vi "Bertta_v09_93.vi"() -> ()   [LabVIEW 2015]
panel:
  out "element":bool
  out "Started:":string
  in  "SHUTDOWN":bool
  in  "MASTER CONTROL":bool
  in  "Tab Control":T1(tab)
  out "Output File":path caption="selected path"
  in  "Browse folder":path=path "" caption="start path"
  in  "Read Seq":bool
  in  "Save Seq":bool
  in  "Configuration file":path=path "C:/Users/shresplab/Desktop/BerttaConfiguration.lvm" caption="Filename"
  in  "OK Button 2":bool
  out "Boolean":bool
  in  "User (initials)":string
  in  "Project name":string
  in  "Description":string
  out "PUMP1":bool
  out "Target amount":dbl
  out "Scale weight":dbl
  out "Amount now":dbl
  out "Flow rate":dbl
  out "Time to target":dbl format="%<%H:%M:%S>t"
  out "Current step":dbl
  out "Target":dbl
  out "Amount now":dbl
  out "Amount now":dbl
  out "Target":dbl
  out "Current step":dbl
  out "Time to target":dbl format="%<%H:%M:%S>t"
  out "Flow rate":dbl
  out "Amount now":dbl
  out "Scale weight":dbl
  out "Target amount":dbl
  out "PUMP2":bool
  out "Sensor OK 6":bool
  out "Sensor OK 5":bool
  out "Sensor OK 4":bool
  out "Sensor OK 3":bool
  in  "OK Button":bool
  in  "Add comment":string
  out "PUMP3":bool
  out "Target amount":dbl
  out "Scale weight":dbl
  out "Amount now":dbl
  out "Flow rate":dbl
  out "Time to target":dbl format="%<%H:%M:%S>t"
  out "Current step":dbl
  out "Target":dbl
  out "Amount now":dbl
  out "Tr":dbl
  out "Tj in":dbl
  out "Tj out":dbl
  out "T set":dbl
  out "Current step":i32
  out "RPM":dbl
  out "Torque 2":dbl
  out "Waveform Chart 5":dynamicdata(graph)
  out "Waveform Chart 6":dynamicdata(graph)
  out "Waveform Chart 7":dynamicdata(graph)
  in  "Tab Control 2":T2(tab)
  out "Waveform Chart 3":dynamicdata(graph)
  out "Waveform Chart 8":dynamicdata(graph)
  out "Waveform Chart 11":dynamicdata(graph)
  out "Waveform Chart 13":dynamicdata(graph)
  out "Waveform Chart 9":dynamicdata(graph)
  out "Table":string[][](table)=[["14.8.2017 18.06.59", "0,000000", "417,670000", "-0,150000", "1,000000", "22,220000", "23,366837", "23,574959", "23,985852", "23,690000", "240,000000", "4,000000", "0,000000", "397,000000", "-397,000000", "1,000000"], ["14.8.2017 18.07.06", "0,000000", "417,640000", "-0,120000", "1,000000", "22,220000", "23,763115", "23,906257", "23,985694", "23,680000", "240,000000", "4,000000", "0,000000", "397,000000", "-397,000000", "1,000000"], ["14.8.2017 18.07.13", "0,000000", "417,640000", "-0,120000", "1,000000", "22,220000", "23,965922", "24,013440", "23,984906", "23,670000", "240,000000", "4,100000", "3,000000", "397,000000", "-397,000000", "1,000000"], ["14.8.2017 18.07.21", "0,000000", "417,640000", "-0,120000", "1,000000", "22,220000", "23,943860", "23,900110", "23,987113", "23,670000", "240,000000", "4,000000", "0,000000", "397,000000", "-397,000000", "1,000000"], ["14.8.2017 18.07.28", "0,000000", "417,640000", "-0,120000", "1,000000", "22,220000", "23,736328", "23,600018", "23,989004", "23,660000", "240,000000", "4,000000", "0,000000", "397,000000", "-397,000000", "1,000000"], ["14.8.2017 18.07.36", "0,000000", "417,640000", "-0,120000", "1,000000", "22,220000", "23,480910", "23,324538", "23,991053", "23,660000", "240,000000", "4,000000", "0,000000", "397,000000", "-397,000000", "1,000000"], ["14.8.2017 18.07.43", "0,000000", "417,640000", "-0,120000", "2,000000", "22,220000", "23,195579", "23,008270", "23,999093", "23,650000", "240,000000", "4,000000", "0,000000", "397,000000", "-397,000000", "1,000000"], ["14.8.2017 18.07.51", "0,000000", "417,650000", "-417,650000", "1,000000", "22,220000", "22,862541", "22,649021", "24,003979", "23,650000", "240,000000", "4,000000", "0,000000", "397,000000", "-397,000000", "2,000000"], ["14.8.2017 18.07.58", "0,000000", "417,640000", "0,010000", "1,000000", "22,220000", "22,541353", "22,354878", "24,005398", "23,650000", "240,000000", "4,000000", "0,000000", "397,000000", "-397,000000", "1,000000"], ["14.8.2017 18.08.06", "0,000000", "417,640000", "0,010000", "1,000000", "22,220000", "22,347931", "22,253738", "24,007605", "23,640000", "240,000000", "4,100000", "0,000000", "397,000000", "-397,000000", "1,000000"], ["14.8.2017 18.08.13", "0,000000", "417,640000", "0,010000", "1,000000", "22,220000", "22,329030", "22,302102", "24,006028", "23,640000", "240,000000", "4,000000", "0,000000", "395,820000", "-395,820000", "1,000000"], ["14.8.2017 18.08.20", "0,000000", "417,640000", "0,010000", "1,000000", "22,220000", "22,466849", "22,511320", "24,002403", "23,630000", "240,000000", "4,000000", "0,000000", "395,830000", "-0,010000", "1,000000"], ["14.8.2017 18.08.28", "0,000000", "417,640000", "0,010000", "1,000000", "22,220000", "22,707062", "22,835101", "24,000984", "23,620000", "240,000000", "4,000000", "0,000000", "395,830000", "-0,010000", "1,000000"], ["14.8.2017 18.08.35", "0,000000", "417,640000", "0,010000", "1,000000", "22,220000", "23,054104", "23,232979", "24,001299", "23,600000", "240,000000", "4,000000", "0,000000", "395,830000", "-0,010000", "1,000000"], ["14.8.2017 18.08.43", "0,000000", "417,640000", "0,010000", "1,000000", "22,220000", "23,412371", "23,522793", "24,002560", "23,590000", "240,000000", "4,000000", "0,000000", "395,820000", "0,000000", "1,000000"], ["14.8.2017 18.08.51", "0,000000", "417,640000", "0,010000", "1,000000", "22,220000", "23,596247", "23,656125", "24,003821", "23,580000", "240,000000", "4,000000", "0,000000", "395,820000", "0,000000", "1,000000"]]
  in  "?":bool
  in  "Time":dbl format="Time to target (min):                %#_g"
  out "Current temp":dbl format="Current temperature (S1):   %#_6g"
  in  "OK Button 3":bool
  in  "T ext / T ext 2":enum32{"Sensor 1", "Sensor 2"}(radio)
  out "Sensor OK":bool
  in  "T fail":dbl=20.0 format="Failsafe temperature:              %#_g"
  in  "Setpoint":dbl=20.0 format="Temperature target:                %#_6g"
  in  "Manual select":T3(radio)
  out "Waveform Chart":dynamicdata(graph)
  out "T external 2":dbl format="Current temperature (S2):    %#_g"
  in  "UPDATE TEMP":bool
  out "Led11 5":bool
  out "RPM":dbl format="%_4f"
  out "Led10 3":bool
  out "Led9 3":bool
  out "Led8 3":bool
  out "Led7 3":bool
  out "Led6 3":bool
  out "Led5 3":bool
  out "Led4 3":bool
  out "Led3 3":bool
  out "Led2 3":bool
  out "Led1 3":bool
  in  "PumpSeq 4":dbl[][](array[numeric])=[[0.0, 0.0, 0.0, 0.0, 0.0, 0.0, 0.0, 0.0, 0.0, 0.0], [0.0, 0.0, 0.0, 0.0, 0.0, 0.0, 0.0, 0.0, 0.0, 0.0], [0.0, 0.0, 0.0, 0.0, 0.0, 0.0, 0.0, 0.0, 0.0, 0.0], [0.0, 0.0, 0.0, 0.0, 0.0, 0.0, 0.0, 0.0, 0.0, 0.0], [0.0, 0.0, 0.0, 0.0, 0.0, 0.0, 0.0, 0.0, 0.0, 0.0], [0.0, 0.0, 0.0, 0.0, 0.0, 0.0, 0.0, 0.0, 0.0, 0.0], [0.0, 0.0, 0.0, 0.0, 0.0, 0.0, 0.0, 0.0, 0.0, 0.0], [0.0, 0.0, 0.0, 0.0, 0.0, 0.0, 0.0, 0.0, 0.0, 0.0], [0.0, 0.0, 0.0, 0.0, 0.0, 0.0, 0.0, 0.0, 0.0, 0.0], [0.0, 0.0, 0.0, 0.0, 0.0, 0.0, 0.0, 0.0, 0.0, 0.0]]
  in  "?":bool
  out "Flow rate (g/min)":dbl
  out "Scale reading":dbl
  out "Step amount now":dbl
  in  "Grams / min":dbl
  out "Waveform Chart 14":dynamicdata(graph)
  in  "?":bool
  out "Total amount now":dbl
  out "Led11 4":bool
  in  "Reset 5":bool
  out "Elapsed / step":i32
  out "Time to target":dbl format="%<%H:%M:%S>t"
  in  "OK Button 4":bool
  out "Led11":bool
  out "RPM":dbl format="%_4f"
  out "Led10":bool
  out "Led9":bool
  out "Led8":bool
  out "Led7":bool
  out "Led6":bool
  out "Led5":bool
  out "Led4":bool
  out "Led3":bool
  out "Led2":bool
  out "Led1":bool
  in  "PumpSeq 2":dbl[][](array[numeric])=[[0.0, 0.0, 0.0, 0.0, 0.0, 0.0, 0.0, 0.0, 0.0, 0.0], [0.0, 0.0, 0.0, 0.0, 0.0, 0.0, 0.0, 0.0, 0.0, 0.0], [0.0, 0.0, 0.0, 0.0, 0.0, 0.0, 0.0, 0.0, 0.0, 0.0], [0.0, 0.0, 0.0, 0.0, 0.0, 0.0, 0.0, 0.0, 0.0, 0.0], [0.0, 0.0, 0.0, 0.0, 0.0, 0.0, 0.0, 0.0, 0.0, 0.0], [0.0, 0.0, 0.0, 0.0, 0.0, 0.0, 0.0, 0.0, 0.0, 0.0], [0.0, 0.0, 0.0, 0.0, 0.0, 0.0, 0.0, 0.0, 0.0, 0.0], [0.0, 0.0, 0.0, 0.0, 0.0, 0.0, 0.0, 0.0, 0.0, 0.0], [0.0, 0.0, 0.0, 0.0, 0.0, 0.0, 0.0, 0.0, 0.0, 0.0], [0.0, 0.0, 0.0, 0.0, 0.0, 0.0, 0.0, 0.0, 0.0, 0.0]]
  in  "?":bool
  out "Flow rate (g/min)":dbl
  out "Scale reading":dbl
  out "Step amount now":dbl
  in  "Grams / min":dbl
  out "Waveform Chart 10":dynamicdata(graph)
  in  "?":bool
  out "Total amount now":dbl
  out "Led11":bool
  in  "Reset 3":bool
  out "Elapsed / step":i32
  out "Time to target":dbl format="%<%H:%M:%S>t"
  in  "OK Button 5":bool
  out "Led11 3":bool
  out "RPM":dbl format="%_4f"
  out "Led10 2":bool
  out "Led9 2":bool
  out "Led8 2":bool
  out "Led7 2":bool
  out "Led6 2":bool
  out "Led5 2":bool
  out "Led4 2":bool
  out "Led3 2":bool
  out "Led2 2":bool
  out "Led1 2":bool
  in  "PumpSeq 3":dbl[][](array[numeric])=[[0.0, 0.0, 0.0, 0.0, 0.0, 0.0, 0.0, 0.0, 0.0, 0.0], [0.0, 0.0, 0.0, 0.0, 0.0, 0.0, 0.0, 0.0, 0.0, 0.0], [0.0, 0.0, 0.0, 0.0, 0.0, 0.0, 0.0, 0.0, 0.0, 0.0], [0.0, 0.0, 0.0, 0.0, 0.0, 0.0, 0.0, 0.0, 0.0, 0.0], [0.0, 0.0, 0.0, 0.0, 0.0, 0.0, 0.0, 0.0, 0.0, 0.0], [0.0, 0.0, 0.0, 0.0, 0.0, 0.0, 0.0, 0.0, 0.0, 0.0], [0.0, 0.0, 0.0, 0.0, 0.0, 0.0, 0.0, 0.0, 0.0, 0.0], [0.0, 0.0, 0.0, 0.0, 0.0, 0.0, 0.0, 0.0, 0.0, 0.0], [0.0, 0.0, 0.0, 0.0, 0.0, 0.0, 0.0, 0.0, 0.0, 0.0], [0.0, 0.0, 0.0, 0.0, 0.0, 0.0, 0.0, 0.0, 0.0, 0.0]]
  in  "?":bool
  out "Flow rate (g/min)":dbl
  out "Scale reading":dbl
  out "Step amount now":dbl
  in  "Grams / min":dbl
  out "Waveform Chart 12":dynamicdata(graph)
  in  "?":bool
  out "Total amount now":dbl
  out "Led11 2":bool
  in  "Reset 4":bool
  out "Elapsed / step":i32
  out "Time to target":dbl format="%<%H:%M:%S>t"
  in  "OK Button 6":bool
  in  "Bypass select 2":enum32{"Remote", "Manual"}(radio)=enum."Manual"
  in  "Port":dbl=13.0
  out "RPM":dbl
  out "Torque":dbl
  in  "Set RPM":dbl(slide) scale=0.0..2000.0
  out "Waveform Chart 4":dynamicdata(graph)
  in  "OK Button 7":bool
  out "PortDev out":dbl[](array[numeric])
  in  "Save PortDev":bool
  out "PortDev in":dbl[](array[numeric])
  in  "dev1":i32
  in  "dev2":i32
  in  "dev3":i32
  in  "dev4":i32
  in  "dev5":i32
  in  "dev6":i32
  in  "dev8":i32
  in  "port1":i32
  in  "port2":i32
  in  "port3":i32
  in  "port4":i32
  in  "port5":i32
  in  "port6":i32
  in  "port7":i32
  in  "port8":i32
  in  "dev7":i32
  in  "Treshold (T/C)":dbl=0.5
  out "DAQ 9217 (PT100)":errorcluster
  out "Config File":dbl[][](array[numeric])
  # "Temperature sensor:"
  # "Manual control:"
  # "PUMP & SCALE 1"
  # "STEP"
  # "TOTAL"
  # "PUMP & SCALE 2"
  # "STEP"
  # "TOTAL"
  # "PUMP & SCALE 3"
  # "STEP"
  # "TOTAL"
  # "Temperature control parameter"
  # "Secondary temperature sensor"
  # "Grams    /   min"
  # "End of sequence"
  # "Manual control"
  # "Grams    /   min"
  # "End of sequence"
  # "Manual control"
  # "Grams    /   min"
  # "End of sequence"
  # "Manual control"
  # "dev1 and dev2 always to port1 and 2\nport1 = port2 = Lauda\n\ndev3 and dev4 always to port3 and port4\nport3 = port4 = Heidolph"
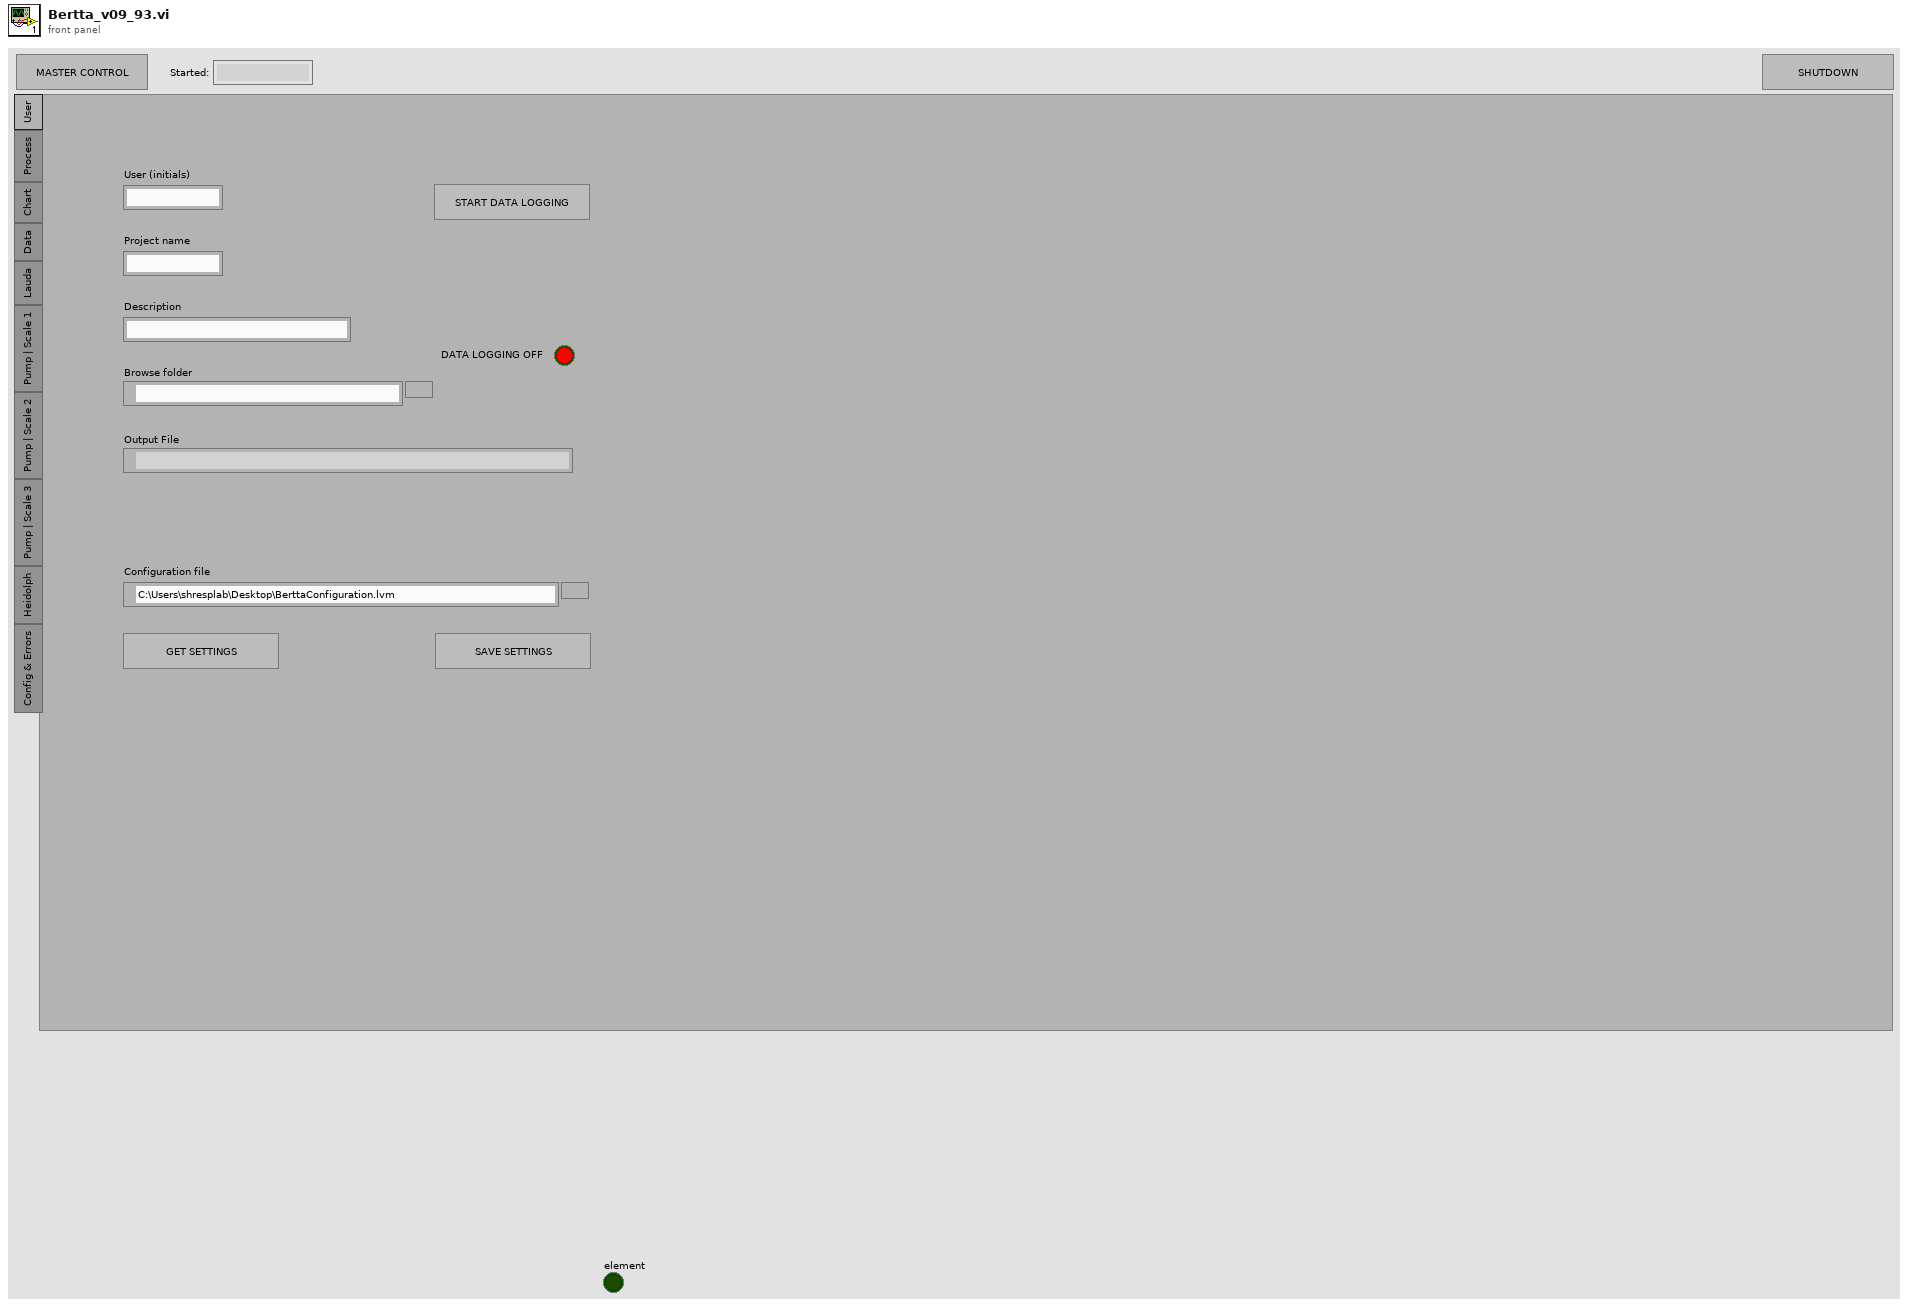
[diagram p1: front panel]
types:
  T1 = enum32{"User", "Process", "Chart", "Data", "Lauda", "Pump | Scale 1", "Pump | Scale 2", "Pump | Scale 3", "Heidolph", "Config & Errors"}
  T2 = enum32{"Temperatures", "Scale / Pump 1", "Scale / Pump 2", "Scale / Pump 3", "RPM / torque"}
  T3 = enum32{"Reactor temperature", "Jacket temperature"}
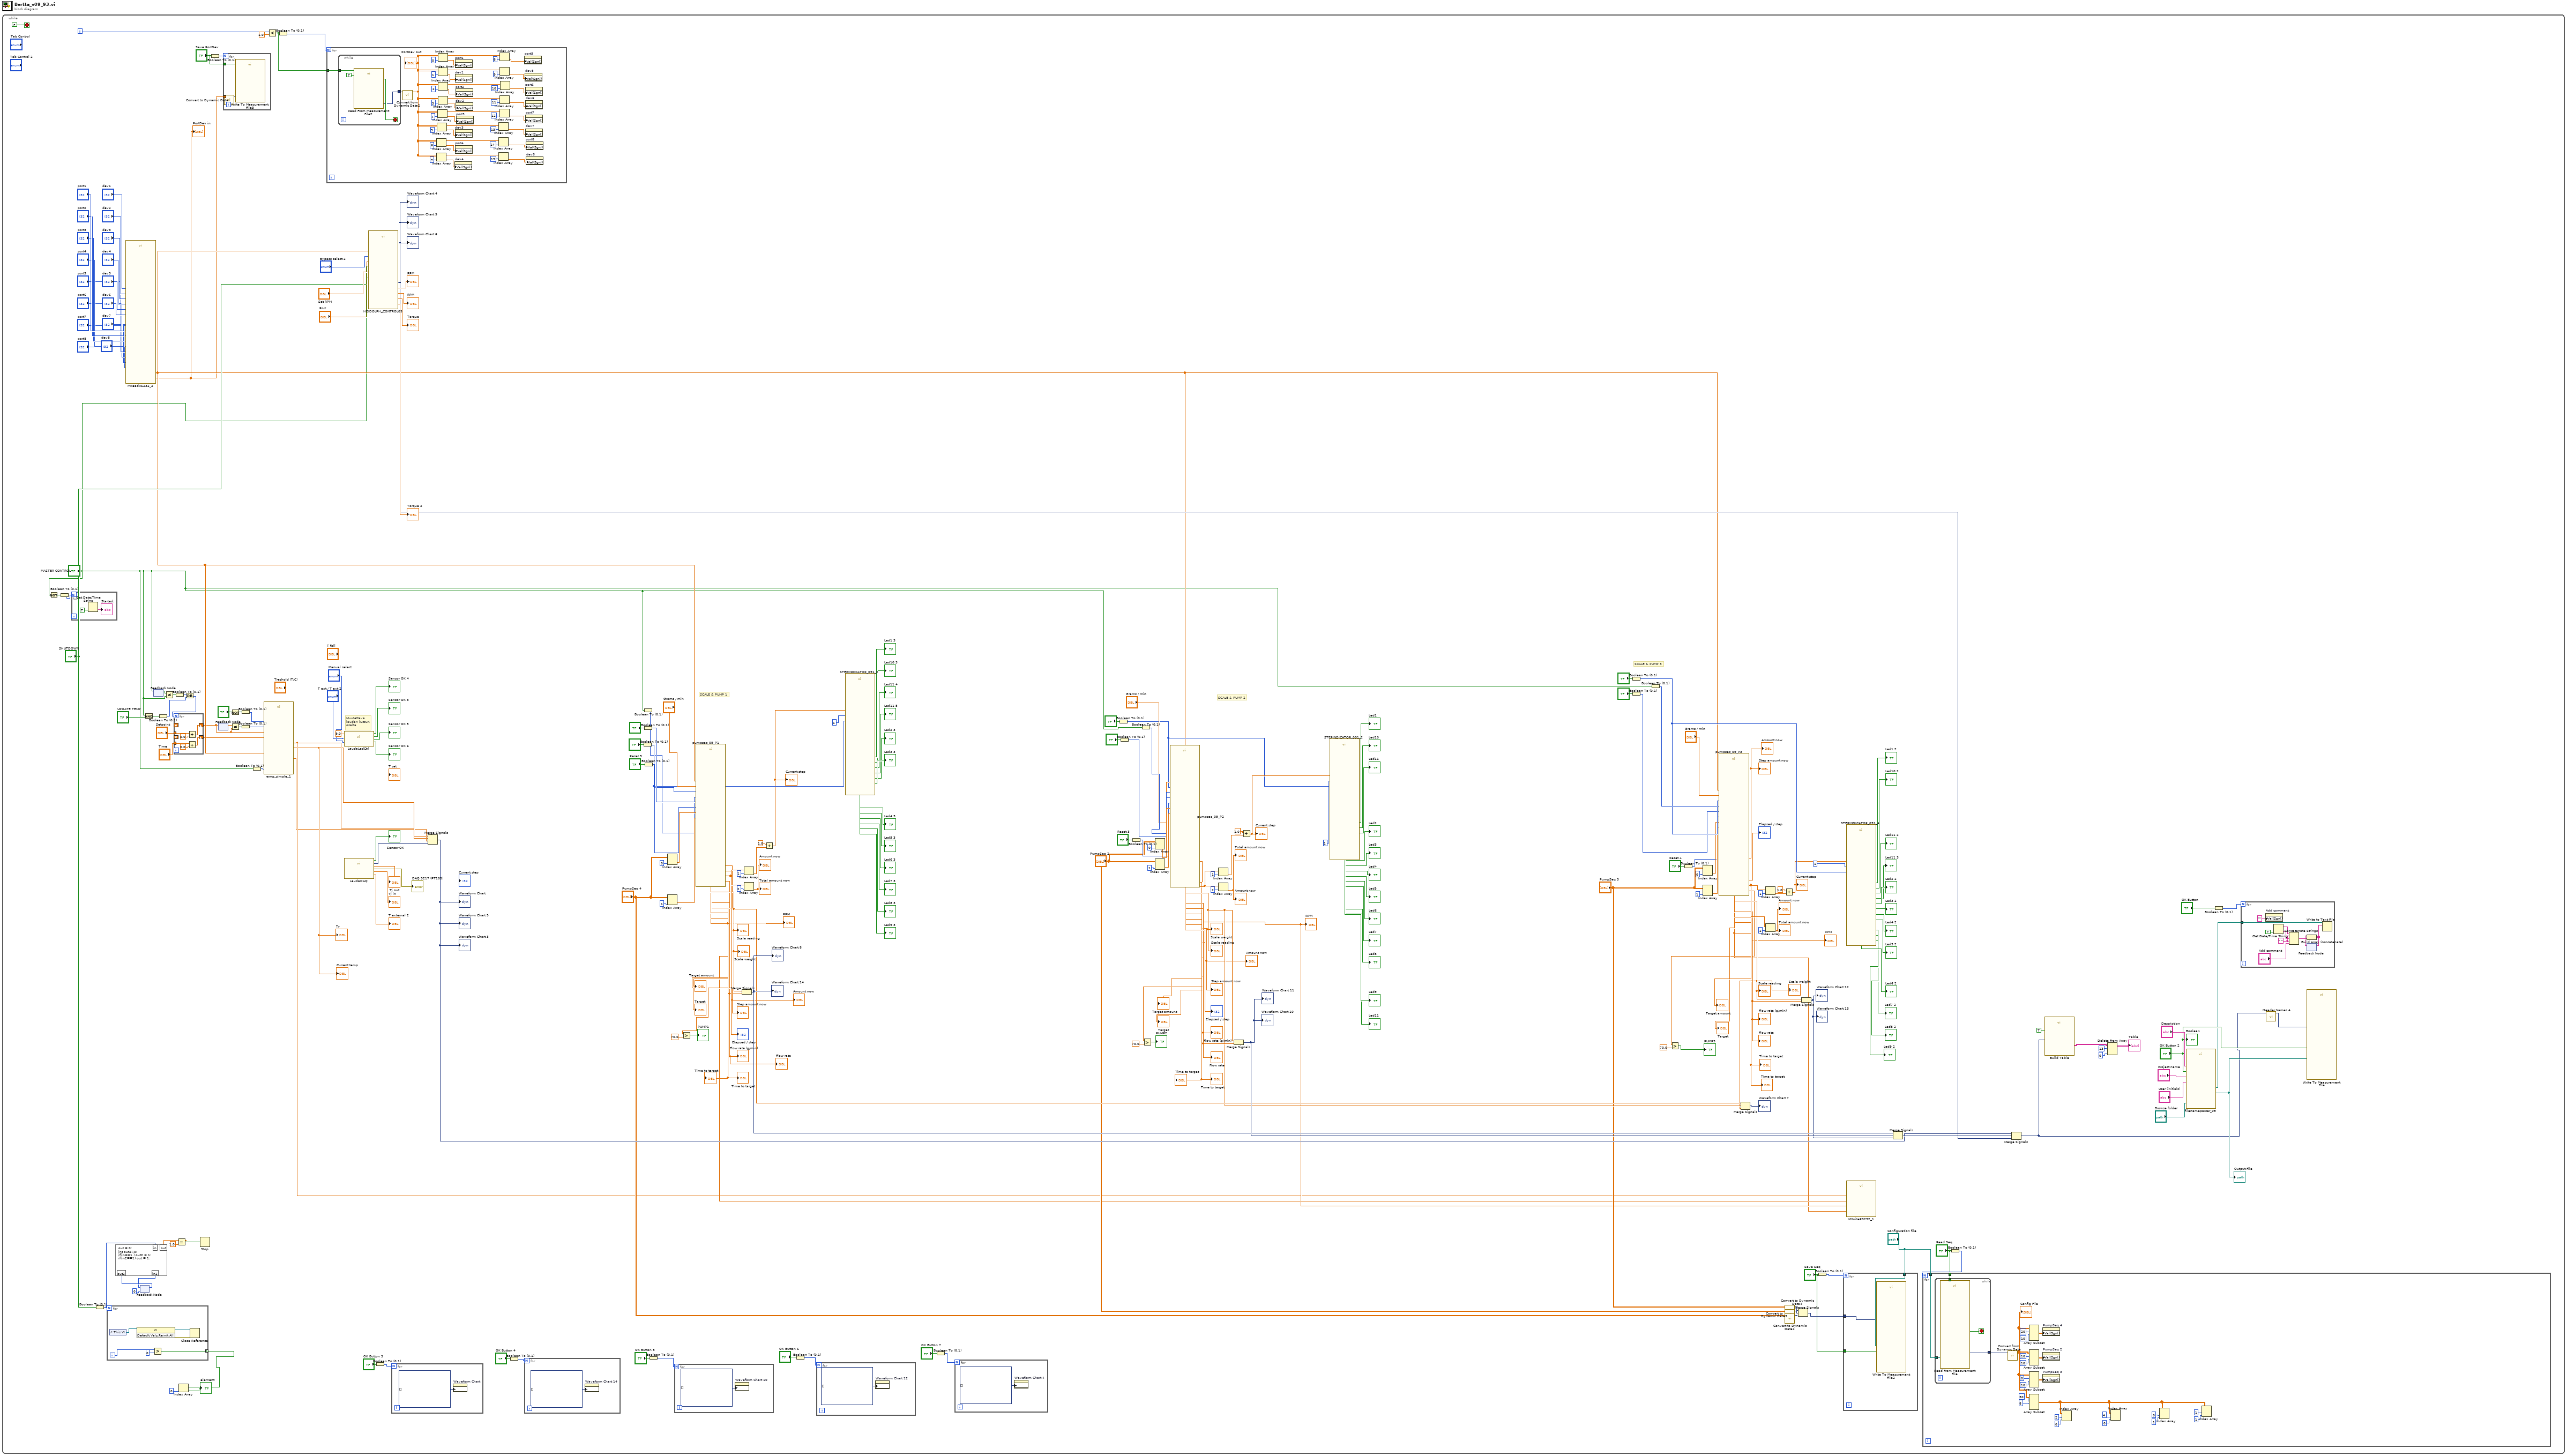
[diagram p0: block diagram]
diagram:
  n1 = while {
    i -> [w5]
    stop <- FALSE stop-if-true
    # "Muutettava\nlaudan kutsun \nosalta"
    # "SCALE & PUMP 1"
    # "SCALE & PUMP 3"
    # "SCALE & PUMP 2"
    n2 = Not(x="MASTER CONTROL") -> (.not. x?=w243:bool)
    n3 = Boolean To (0,1)(Boolean=w243) -> (0, 1=w244:i16)
    n4 = for {
      N: w244 -> [_]
      n5 = Get Date/Time String(want seconds? (F)=TRUE) -> (time string=→"Started:":string)  [unwired: 2 in, 1 out]
    }
    n6 = Boolean To (0,1)(Boolean="SHUTDOWN") -> (0, 1=w227:i16)
    n7 = for {
      N: w227 -> [_]
      tunnel: [w349] -> w242 mode=indexing
      i -> [w351]
      n8 = control-ref of="This VI"() -> (w354:refnum<vi>)
      n9 = invoke class="VI" method="Default Vals.Reinit All"(reference=w354) -> (reference out=w352:refnum<vi>, error out=w353:errorcluster)  [unwired: 2 in, 1 out]
      n10 = Greater?(x=w351, y=0) -> (0:w349:bool)
      n11 = Close Reference(reference=w352, error in (no error)=w353) -> ()  [unwired: 1 out]
    }
    n12 = call "MReadRS232_2.vi"("port1"="port1", "dev1"="dev1", "port2"="port2", "dev2"="dev2", "port3"="port3", "dev7"="dev7", "dev8"="dev8", "port7"="port7", "port8"="port8", "dev5"="dev5", "port5"="port5", "dev4"="dev4", "dev6"="dev6", "port6"="port6", "port4"="port4", "dev3"="dev3") -> ("output array"=w9:dbl[], "params"=w48:dbl[])  [unwired: 2 in]
    "PortDev in" <- w9
    n13 = feedback #1(0) -> (w225:i32)
    n14 = formula code="out = 0;\nint out2=0;\nif(in==1 ) out2 = 1;\nif(in2==1) out = 1;"("in"=w227, "in2"=w225) -> ("out"=w229:dbl, "out2"=w226:i32)
    n15 = feedback-in #1(w226) -> ()
    n16 = And(x="MASTER CONTROL", y="UPDATE TEMP") -> (x .and. y?=w40:bool)
    n17 = feedback #2() -> (w31:bool)  [unwired: 1 in]
    n18 = feedback-in #2("MASTER CONTROL") -> ()
    n19 = Boolean To (0,1)(Boolean=w40) -> (0, 1=w28:i16)
    n20 = Not Equal?(x=w31, y="MASTER CONTROL") -> (x != y?=w30:bool)
    n21 = Boolean To (0,1)(Boolean=w30) -> (0, 1=w27:i16)
    n22 = Equal?(x=w229, y=1.0) -> (x = y?=w228:bool)
    n23 = Index Array(array=w242, index=0) -> (element=→"element":bool)
    n24 = Or(x=w27, y=w28) -> (x .or. y?=w26:i16)
    n25 = for {
      N: w26 -> [_]
      tunnel: "Time" -> [w301]
      shift-right: [w300] -> w42
      shift-left: _ -> [_]
      tunnel: "Setpoint" -> [w298]
      shift-right: [w297] -> w38
      shift-left: _ -> [_]
      n26 = Add(x=w298, y=0.0) -> (x+y=w297:dbl)
      n27 = Add(x=w301, y=0.0) -> (x+y=w300:dbl)
    }
    n28 = Stop(stop? (T)=w228) -> ()
    n29 = Boolean To (0,1)(Boolean="Save PortDev") -> (0, 1=w8:i16)
    n30 = feedback-in #3(w38) -> ()
    n31 = feedback #3() -> (w39:dbl)  [unwired: 1 in]
    n32 = for {
      N: w8 -> [_]
      tunnel: w9 -> [w296]
      tunnel: "Save PortDev" -> [w294]
      n33 = call "Convert to Dynamic Data"("Array"=w296) -> ("Dynamic Data Type"=w295:dynamicdata)  [unwired: 3 in]
      n34 = call "Write To Measurement File3"("Signals"=w295, "Reset"=w294) -> ()  [unwired: 15 in, 3 out]
    }
    n35 = Not(x="?") -> (.not. x?=w34:bool)
    n36 = Not Equal?(x=w39, y=w38) -> (x != y?=w37:bool)
    n37 = Boolean To (0,1)(Boolean=w34) -> (0, 1=w36:i16)
    n38 = Boolean To (0,1)(Boolean=w37) -> (0, 1=w32:i16)
    n39 = Boolean To (0,1)(Boolean="MASTER CONTROL") -> (0, 1=w33:i16)
    n40 = call "ramp_simple_1.vi"("array"=w48, "time_set"=w42, "T_sp"=w38, "master"=w33, "reset"=w32, "pause"=w36) -> ("T control"=w47:dbl, "Tr"=w46:dbl, "Tin"=w45:dbl)  [unwired: 2 in, 1 out]
    "Tr" <- w46
    "Current temp" <- w46
    n41 = Less?(x=w5, y=1.0) -> (x < y?=w3:bool)
    n42 = Boolean To (0,1)(Boolean=w3) -> (0, 1=w4:i16)
    n43 = for {
      N: w4 -> [_]
      tunnel: w3 -> [w289]
      n44 = while {
        tunnel: [w292] -> w288
        tunnel: w289 -> [w290]
        stop <- w293 stop-if-true
        n45 = call "Read From Measurement File2"("Enable"=TRUE, "Reset"=w290) -> ("Signals"=w292:dynamicdata, "EOF?"=w293:bool)  [unwired: 4 in, 4 out]
      }
      n46 = call "Convert from Dynamic Data2"("Dynamic Data Type"=w288) -> ("Array"=w271:dbl[])  [unwired: 3 in]
      "PortDev out" <- w271
      n47 = Index Array(array=w271, index=6) -> (element=w264:dbl)
      n48 = Index Array(array=w271, index=7) -> (element=w263:dbl)
      n49 = Index Array(array=w271, index=5) -> (element=w265:dbl)
      n50 = Index Array(array=w271, index=4) -> (element=w266:dbl)
      n51 = Index Array(array=w271, index=0) -> (element=w270:dbl)
      n52 = Index Array(array=w271, index=1) -> (element=w269:dbl)
      n53 = Index Array(array=w271, index=3) -> (element=w267:dbl)
      n54 = Index Array(array=w271, index=2) -> (element=w268:dbl)
      n55 = property on="dev4" class="DigNum (strict)"("Val(Sgnl)"=w263) -> ()  [unwired: 2 in, 2 out]
      n56 = property on="dev3" class="DigNum (strict)"("Val(Sgnl)"=w265) -> ()  [unwired: 2 in, 2 out]
      n57 = property on="port4" class="DigNum (strict)"("Val(Sgnl)"=w264) -> ()  [unwired: 2 in, 2 out]
      n58 = property on="port1" class="DigNum (strict)"("Val(Sgnl)"=w270) -> ()  [unwired: 2 in, 2 out]
      n59 = property on="dev1" class="DigNum (strict)"("Val(Sgnl)"=w269) -> ()  [unwired: 2 in, 2 out]
      n60 = property on="port2" class="DigNum (strict)"("Val(Sgnl)"=w268) -> ()  [unwired: 2 in, 2 out]
      n61 = property on="dev2" class="DigNum (strict)"("Val(Sgnl)"=w267) -> ()  [unwired: 2 in, 2 out]
      n62 = property on="port3" class="DigNum (strict)"("Val(Sgnl)"=w266) -> ()  [unwired: 2 in, 2 out]
      n63 = Index Array(array=w271, index=14) -> (element=w256:dbl)
      n64 = Index Array(array=w271, index=15) -> (element=w255:dbl)
      n65 = Index Array(array=w271, index=13) -> (element=w257:dbl)
      n66 = Index Array(array=w271, index=12) -> (element=w258:dbl)
      n67 = Index Array(array=w271, index=8) -> (element=w262:dbl)
      n68 = Index Array(array=w271, index=9) -> (element=w261:dbl)
      n69 = Index Array(array=w271, index=11) -> (element=w259:dbl)
      n70 = Index Array(array=w271, index=10) -> (element=w260:dbl)
      n71 = property on="port5" class="DigNum (strict)"("Val(Sgnl)"=w262) -> ()  [unwired: 2 in, 2 out]
      n72 = property on="dev5" class="DigNum (strict)"("Val(Sgnl)"=w261) -> ()  [unwired: 2 in, 2 out]
      n73 = property on="port6" class="DigNum (strict)"("Val(Sgnl)"=w260) -> ()  [unwired: 2 in, 2 out]
      n74 = property on="dev6" class="DigNum (strict)"("Val(Sgnl)"=w259) -> ()  [unwired: 2 in, 2 out]
      n75 = property on="port7" class="DigNum (strict)"("Val(Sgnl)"=w258) -> ()  [unwired: 2 in, 2 out]
      n76 = property on="dev7" class="DigNum (strict)"("Val(Sgnl)"=w257) -> ()  [unwired: 2 in, 2 out]
      n77 = property on="port8" class="DigNum (strict)"("Val(Sgnl)"=w256) -> ()  [unwired: 2 in, 2 out]
      n78 = property on="dev8" class="DigNum (strict)"("Val(Sgnl)"=w255) -> ()  [unwired: 2 in, 2 out]
    }
    n79 = call "LaudaLedCtrl.vi"("Manual select"="Manual select", "T ext / T ext in"="T ext / T ext 2", "Lauda port"=9.0) -> ("Sensor OK 5"=→"Sensor OK 5":bool, "Sensor OK 3"=→"Sensor OK 3":bool, "Sensor OK 4"=→"Sensor OK 4":bool, "Sensor OK 6"=→"Sensor OK 6":bool)  [unwired: 5 in]
    n80 = call "LaudaDAQ.vi"() -> ("error out"=→"DAQ 9217 (PT100)":errorcluster, 1:"Tj out"=→"Tj out":dbl, "data"=w116:dynamicdata, "Sensor OK"=→"Sensor OK":bool, 4:"Tj out"=→"Tj in":dbl, "T external 2"=→"T external 2":dbl)  [unwired: 6 in]
    n81 = call "HEIDOLPH_CONTROL09.vi"("master"="MASTER CONTROL", "Array"=w48, "shutdown"="SHUTDOWN", "Bypass select"="Bypass select 2", "Set RPM"="Set RPM", "Device port"="Port") -> ("Dynamic Data"=w117:dynamicdata, "RPM"=→"RPM":dbl, "RPM 2"=→"RPM":dbl, "Torque"=→"Torque":dbl, "Torque 2"=→"Torque 2":dbl)  [unwired: 1 in]
    "Waveform Chart 4" <- w117
    "Waveform Chart 6" <- w117
    "Waveform Chart 9" <- w117
    n82 = Boolean To (0,1)(Boolean="OK Button 3") -> (0, 1=w59:i16)
    n83 = for {
      N: w59 -> [_]
      n84 = property on="Waveform Chart" class="WFChart (strict)"("History Data"=dynamicdata[] []) -> ()  [unwired: 2 in, 2 out]
    }
    n85 = Merge Signals(w47, w46, w45, w116) -> (w118:dynamicdata)
    "Waveform Chart 3" <- w118
    "Waveform Chart" <- w118
    "Waveform Chart 5" <- w118
    n86 = Boolean To (0,1)(Boolean="OK Button 4") -> (0, 1=w57:i16)
    n87 = for {
      N: w57 -> [_]
      n88 = property on="Waveform Chart 14" class="WFChart (strict)"("History Data"=dynamicdata[] []) -> ()  [unwired: 2 in, 2 out]
    }
    n89 = Boolean To (0,1)(Boolean="?") -> (0, 1=w126:i16)
    n90 = Boolean To (0,1)(Boolean="?") -> (0, 1=w130:i16)
    n91 = Boolean To (0,1)(Boolean="MASTER CONTROL") -> (0, 1=w122:i16)
    n92 = Boolean To (0,1)(Boolean="Reset 5") -> (0, 1=w129:i16)
    n93 = Boolean To (0,1)(Boolean="OK Button 5") -> (0, 1=w55:i16)
    n94 = Index Array(array="PumpSeq 4", index (col)=0) -> (element=w134:dbl[])  [unwired: 1 in]
    n95 = Index Array(array="PumpSeq 4", index (col)=1) -> (element=w155:dbl[])  [unwired: 1 in]
    n96 = for {
      N: w55 -> [_]
      n97 = property on="Waveform Chart 10" class="WFChart (strict)"("History Data"=dynamicdata[] []) -> ()  [unwired: 2 in, 2 out]
    }
    n98 = call "pumpsec_09_P1.vi"("reset"=w129, "master"=w122, "manual"=w126, "pause"=w130, "Array"=w48, "Target"=w134, "fr_manual"="Grams / min", "Time"=w155) -> ("pumpCtrl"=w100:dbl, "totaltarget"=→"Target":dbl, "target_step"=→"Target amount":dbl, "REGLO D"=w66:dbl, "time_to_target"=→"Time to target" →"Time to target":dbl, "step_fr"=w77:dbl, "amount_step"=→"Amount now" →"Step amount now":dbl, "Scale"=w112:dbl, "elapsed_step"=→"Elapsed / step":dbl, "params"=w152:dbl[])  [unwired: 8 in, 2 out]
    "Flow rate" <- w77
    "Scale weight" <- w112
    "Scale reading" <- w112
    "Flow rate (g/min)" <- w77
    "RPM" <- w66
    n99 = Greater?(x=w100, y=70.0) -> (0:→"PUMP1":bool)
    n100 = Merge Signals(w112, w77) -> (w121:dynamicdata)
    "Waveform Chart 8" <- w121
    "Waveform Chart 14" <- w121
    n101 = Index Array(array=w152, index=1) -> (element=w149:dbl)
    n102 = Index Array(array=w152, index=2) -> (element=→"Amount now" →"Total amount now":dbl)
    n103 = Add(x=1.0, y=w149) -> (x+y=w78:dbl)
    "Current step" <- w78
    n104 = Boolean To (0,1)(Boolean="OK Button 6") -> (0, 1=w53:i16)
    n105 = for {
      N: w53 -> [_]
      n106 = property on="Waveform Chart 12" class="WFChart (strict)"("History Data"=dynamicdata[] []) -> ()  [unwired: 2 in, 2 out]
    }
    n107 = call "STEPINDICATOR_091_2.vi"("current step"=w78, "enable"=i16 1, "manual"=w126) -> ("Led 8"=→"Led8 3":bool, "Led 10"=→"Led10 3":bool, "Led 11"=→"Led11 4":bool, "Led 7"=→"Led7 3":bool, "Led 1"=→"Led1 3":bool, "Led 6"=→"Led6 3":bool, "Led 2"=→"Led2 3":bool, "Led 12"=→"Led11 5":bool, "Led 5"=→"Led5 3":bool, "Led 4"=→"Led4 3":bool, "Led 3"=→"Led3 3":bool, "Led 9"=→"Led9 3":bool)  [unwired: 1 in]
    n108 = Boolean To (0,1)(Boolean="OK Button 7") -> (0, 1=w51:i16)
    n109 = for {
      N: w51 -> [_]
      n110 = property on="Waveform Chart 4" class="WFChart (strict)"("History Data"=dynamicdata[] []) -> ()  [unwired: 2 in, 2 out]
    }
    n111 = Boolean To (0,1)(Boolean="?") -> (0, 1=w189:i16)
    n112 = Boolean To (0,1)(Boolean="?") -> (0, 1=w216:i16)
    n113 = Boolean To (0,1)(Boolean="Reset 3") -> (0, 1=w214:i16)
    n114 = Boolean To (0,1)(Boolean="MASTER CONTROL") -> (0, 1=w208:i16)
    n115 = Index Array(array="PumpSeq 2", index (col)=0 ("disabled index (col)")) -> (element=w219:dbl[])  [unwired: 1 in]
    n116 = Index Array(array="PumpSeq 2", index (col)=1 ("disabled index (col)")) -> (element=w218:dbl[])  [unwired: 1 in]
    n117 = call "pumpsec_09_P2.vi"("reset"=w214, "master"=w208, "manual"=w189, "pause"=w216, "Array"=w48, "Target"=w219, "fr_manual"="Grams / min", "Time"=w218) -> ("pumpCtrl"=w96:dbl, "totaltarget"=→"Target":dbl, "target_step"=→"Target amount":dbl, "REGLO D"=w65:dbl, "time_to_target"=→"Time to target" →"Time to target":dbl, "step_fr"=w115:dbl, "amount_step"=→"Amount now" →"Step amount now":dbl, "Scale"=w111:dbl, "elapsed_step"=→"Elapsed / step":dbl, "params"=w209:dbl[])  [unwired: 8 in, 2 out]
    "Scale weight" <- w111
    "Flow rate" <- w115
    "Scale reading" <- w111
    "Flow rate (g/min)" <- w115
    "RPM" <- w65
    n118 = Greater?(x=w96, y=70.0) -> (0:→"PUMP2":bool)
    n119 = Index Array(array=w209, index=1) -> (element=w212:dbl)
    n120 = Index Array(array=w209, index=2) -> (element=→"Amount now" →"Total amount now":dbl)
    n121 = Merge Signals(w111, w115) -> (w123:dynamicdata)
    "Waveform Chart 11" <- w123
    "Waveform Chart 10" <- w123
    n122 = Add(x=1.0, y=w212) -> (x+y=w206:dbl)
    "Current step" <- w206
    n123 = call "STEPINDICATOR_091_2.vi"("current step"=w206, "enable"=i16 1, "manual"=w189) -> ("Led 8"=→"Led8":bool, "Led 10"=→"Led10":bool, "Led 11"=→"Led11":bool, "Led 7"=→"Led7":bool, "Led 1"=→"Led1":bool, "Led 6"=→"Led6":bool, "Led 2"=→"Led2":bool, "Led 12"=→"Led11":bool, "Led 5"=→"Led5":bool, "Led 4"=→"Led4":bool, "Led 3"=→"Led3":bool, "Led 9"=→"Led9":bool)  [unwired: 1 in]
    n124 = Boolean To (0,1)(Boolean="?") -> (0, 1=w183:i16)
    n125 = Boolean To (0,1)(Boolean="?") -> (0, 1=w182:i16)
    n126 = Boolean To (0,1)(Boolean="MASTER CONTROL") -> (0, 1=w184:i16)
    n127 = Boolean To (0,1)(Boolean="Reset 4") -> (0, 1=w164:i16)
    n128 = Index Array(array="PumpSeq 3", index (col)=0 ("disabled index (col)")) -> (element=w167:dbl[])  [unwired: 1 in]
    n129 = Index Array(array="PumpSeq 3", index (col)=1 ("disabled index (col)")) -> (element=w166:dbl[])  [unwired: 1 in]
    n130 = call "pumpsec_09_P3.vi"("reset"=w164, "master"=w184, "manual"=w183, "pause"=w182, "Array"=w48, "Target"=w167, "fr_manual"="Grams / min", "Time"=w166) -> ("pumpCtrl"=w93:dbl, "totaltarget"=→"Target":dbl, "target_step"=→"Target amount":dbl, "REGLO D"=w64:dbl, "time_to_target"=→"Time to target" →"Time to target":dbl, "step_fr"=w114:dbl, "amount_step"=→"Amount now" →"Step amount now":dbl, "Scale"=w110:dbl, "elapsed_step"=→"Elapsed / step":dbl, "params"=w157:dbl[])  [unwired: 8 in, 2 out]
    "Scale weight" <- w110
    "Flow rate" <- w114
    "Scale reading" <- w110
    "Flow rate (g/min)" <- w114
    "RPM" <- w64
    n131 = Greater?(x=w93, y=70.0) -> (0:→"PUMP3":bool)
    n132 = Merge Signals(w112, w111, w110) -> (→"Waveform Chart 7":dynamicdata)
    n133 = Index Array(array=w157, index=1) -> (element=w158:dbl)
    n134 = Index Array(array=w157, index=2) -> (element=→"Amount now" →"Total amount now":dbl)
    n135 = Add(x=1.0, y=w158) -> (x+y=w156:dbl)
    "Current step" <- w156
    n136 = call "Convert to Dynamic Data4"("2D Array"="PumpSeq 3") -> ("Dynamic Data Type"=w69:dynamicdata)  [unwired: 3 in]
    n137 = call "Convert to Dynamic Data3"("2D Array"="PumpSeq 2") -> ("Dynamic Data Type"=w71:dynamicdata)  [unwired: 3 in]
    n138 = call "Convert to Dynamic Data2"("2D Array"="PumpSeq 4") -> ("Dynamic Data Type"=w74:dynamicdata)  [unwired: 3 in]
    n139 = Merge Signals(w69, w71, w74) -> (w73:dynamicdata)
    n140 = Merge Signals(w110, w114) -> (w120:dynamicdata)
    "Waveform Chart 13" <- w120
    "Waveform Chart 12" <- w120
    n141 = Boolean To (0,1)(Boolean="Save Seq") -> (0, 1=w68:i16)
    n142 = for {
      N: w68 -> [_]
      tunnel: w73 -> [w347]
      tunnel: "Configuration file" -> [w348]
      tunnel: "Save Seq" -> [w346]
      n143 = call "Write To Measurement File2"("Signals"=w347, "Reset"=w346, "Filename"=w348) -> ()  [unwired: 14 in, 3 out]
    }
    n144 = call "STEPINDICATOR_091_4.vi"("current step"=w156, "enable"=i16 1, "manual"=w183) -> ("Led 8"=→"Led8 2":bool, "Led 10"=→"Led10 2":bool, "Led 11"=→"Led11 2":bool, "Led 7"=→"Led7 2":bool, "Led 1"=→"Led1 2":bool, "Led 6"=→"Led6 2":bool, "Led 2"=→"Led2 2":bool, "Led 12"=→"Led11 3":bool, "Led 5"=→"Led5 2":bool, "Led 4"=→"Led4 2":bool, "Led 3"=→"Led3 2":bool, "Led 9"=→"Led9 2":bool)  [unwired: 1 in]
    n145 = call "MWriteRS232_1.vi"("P3"=w64, "P2"=w65, "P1"=w66, "LAUDA"=w47) -> ()  [unwired: 8 in]
    n146 = Merge Signals(w121, w123, w120) -> (w119:dynamicdata)
    n147 = Boolean To (0,1)(Boolean="Read Seq") -> (0, 1=w67:i16)
    n148 = for {
      N: w67 -> [_]
      tunnel: "Configuration file" -> [w319]
      tunnel: "Read Seq" -> [w318]
      n149 = while {
        tunnel: [w345] -> w341
        tunnel: w319 -> [w344]
        tunnel: w318 -> [w342]
        stop <- w343 stop-if-true
        n150 = call "Read From Measurement File"("Filename"=w344, "Reset"=w342) -> ("Signals"=w345:dynamicdata, "EOF?"=w343:bool)  [unwired: 4 in, 4 out]
      }
      n151 = call "Convert from Dynamic Data"("Dynamic Data Type"=w341) -> ("Array"=w331:dbl[][])  [unwired: 3 in]
      "Config File" <- w331
      n152 = Array Subset(array=w331, index (row)=20 ("index"), length (row)=10 ("length")) -> (w338:dbl[][])  [unwired: 2 in]
      n153 = Array Subset(array=w331, index (row)=10 ("index"), length (row)=10 ("length")) -> (w333:dbl[][])  [unwired: 2 in]
      n154 = Array Subset(array=w331, index (row)=0 ("index"), length (row)=10 ("length")) -> (w332:dbl[][])  [unwired: 2 in]
      n155 = Array Subset(array=w331, index (row)=30 ("index"), length (row)=8 ("length")) -> (w320:dbl[][])  [unwired: 2 in]
      n156 = property on="PumpSeq 4" class="Arr (strict)"("Val(Sgnl)"=w338) -> ()  [unwired: 2 in, 2 out]
      n157 = property on="PumpSeq 2" class="Arr (strict)"("Val(Sgnl)"=w333) -> ()  [unwired: 2 in, 2 out]
      n158 = property on="PumpSeq 3" class="Arr (strict)"("Val(Sgnl)"=w332) -> ()  [unwired: 2 in, 2 out]
      n159 = Index Array(array=w320, index (row)=2, index (col)=0 ("disabled index (col)")) -> ()  [unwired: 1 out]
      n160 = Index Array(array=w320, index (row)=4, index (col)=0 ("disabled index (col)")) -> ()  [unwired: 1 out]
      n161 = Index Array(array=w320, index (row)=0, index (col)=1 ("disabled index (col)")) -> ()  [unwired: 1 out]
      n162 = Index Array(array=w320, index (row)=1, index (col)=1 ("disabled index (col)")) -> ()  [unwired: 1 out]
    }
    n163 = Merge Signals(w118, w119, w117) -> (w1:dynamicdata)
    n164 = call "Build Table"("Include time data"=TRUE, "Signals"=w1) -> ("Table"=w237:string[][])  [unwired: 3 in, 6 out]
    n165 = Delete From Array(array=w237, length=13, index (col)=0 ("index (row)")) -> (array with subset deleted=→"Table":string[][])  [unwired: 1 in, 1 out]
    n166 = call "filenameparser_09.vi"("Description"="Description", "start path"="Browse folder", "Project name"="Project name", "User (initials)"="User (initials)", "OK Button in"="OK Button 2") -> ("appended path 2"=w49:path, "appended path"=w233:path)  [unwired: 4 in, 1 out]
    "Output File" <- w49
    n167 = Boolean To (0,1)(Boolean="OK Button") -> (0, 1=w232:i16)
    n168 = for {
      N: w232 -> [_]
      tunnel: w233 -> [w310]
      w314 = " " ("string")
      n169 = property on="Add comment" class="Str"("Val(Sgnl)"="" ("Value (Signaling)")) -> ()  [unwired: 2 in, 2 out]
      n170 = Get Date/Time String(want seconds? (F)=TRUE) -> (date string=w317:string, time string=w315:string)  [unwired: 2 in]
      n171 = Concatenate Strings(w317, w314, w315, w314, "Add comment") -> (w313:string)
      n172 = feedback #4() -> (w312:string[])  [unwired: 1 in]
      n173 = Build Array (concatenate)(w312, w313) -> (w311:string[])
      n174 = feedback-in #4(w311) -> ()
      n175 = Write to Text File(file (use dialog)=w310, text=w311) -> ()  [unwired: 2 in, 3 out]
    }
    n176 = call "Header Names 4.vi"("Dynamic Data"=w1) -> ("Signals Out"=w2:dynamicdata)  [unwired: 10 in]
    n177 = call "Write To Measurement File"("Signals"=w2, "Enable"="OK Button 2", "Filename"=w49) -> ()  [unwired: 14 in, 3 out]
    "Boolean" <- "OK Button 2"
  }
